vi "Write_To_File.vi"(8 "error in (no error)":errorcluster, 10 "Elevator Fleet":T1, 11 "refnum in":refnum<file>) -> (0 "error out":errorcluster, 3 "refnum out":refnum<file>)   [LabVIEW 2026]
uses:
  Controls/Elevator_Fleet.ctl
  Controls/Elevator_Status.ctl
  Controls/Door_Status_Enum.ctl
  Controls/Occupy_Status.ctl
  Controls/Floor_Status.ctl
  Controls/Motion_Status_Enum.ctl
  Controls/Car_Calls_Status.ctl
  Controls/Hall_Calls_Status.ctl
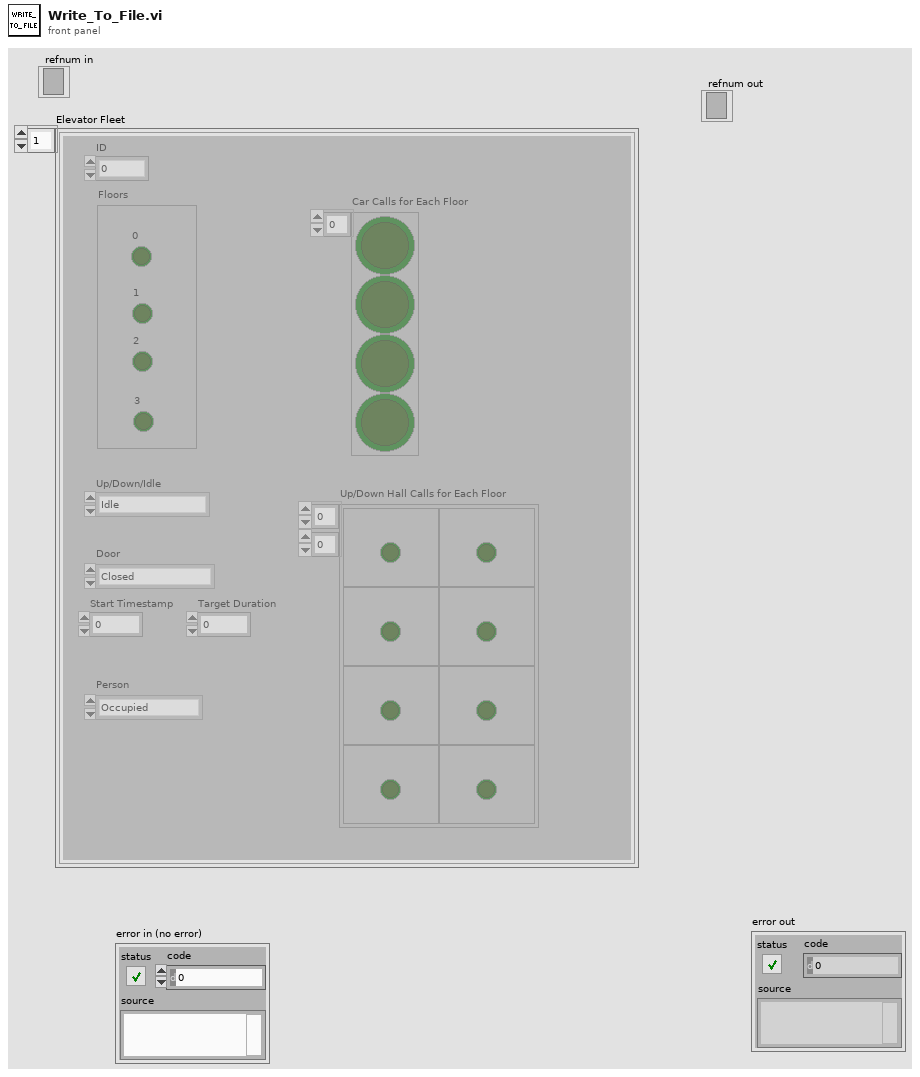
[diagram p1: front panel]
types:
  T1 = typedef "Elevator_Fleet.ctl" = T2[]
  T2 = typedef "Elevator_Status.ctl" = cluster{"Door":T3, "Person":T4, "Floors":T5, "Up/Down/Idle":T6, "Car Calls for Each Floor":T7, "Up/Down Hall Calls for Each Floor":T8, "ID":i32, "Start Timestamp":u32, "Target Duration":dbl}
  T3 = typedef "Door_Status_Enum.ctl" = enum16{"Closed", "Open", "Opening", "Closing"}
  T4 = typedef "Occupy_Status.ctl" = enum16{"Occupied", "Empty"}
  T5 = typedef "Floor_Status.ctl" = cluster{"0":bool, "1":bool, "2":bool, "3":bool}
  T6 = typedef "Motion_Status_Enum.ctl" = enum16{"Idle", "Up", "Down"}
  T7 = typedef "Car_Calls_Status.ctl" = bool[]
  T8 = typedef "Hall_Calls_Status.ctl" = cluster{bool}[][]
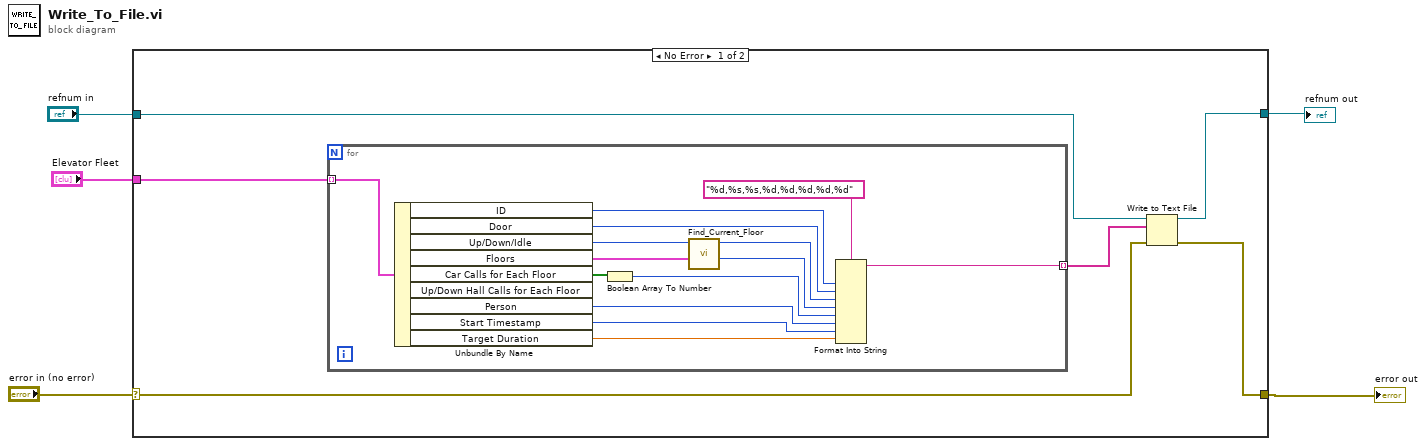
[diagram p0: block diagram]
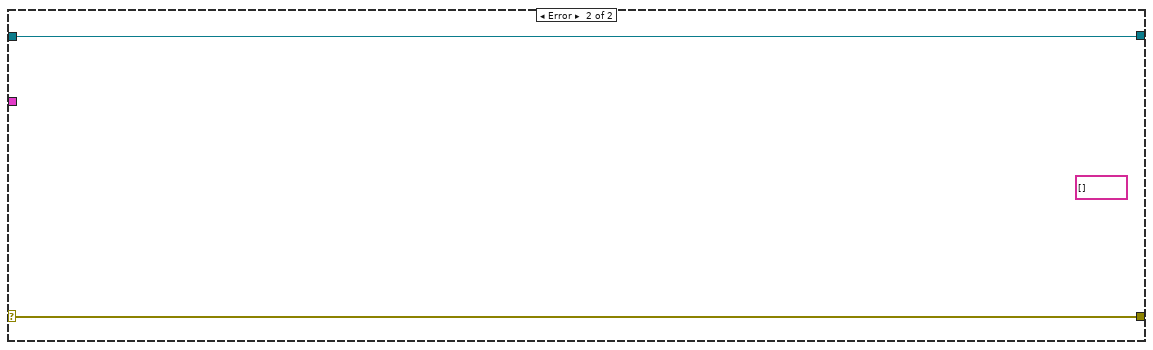
[diagram p2: hidden frame]
diagram:
  n1 = case shown="No Error" "error in (no error)" {
    selector: "error in (no error)" -> [w7 w26]
    tunnel: "Elevator Fleet" -> [w11 _]
    tunnel: [w6 w26] -> w3
    tunnel: "refnum in" -> [w8 w25]
    tunnel: [w10 w25] -> w1
    frame No Error {
      n2 = for {
        tunnel: w11 -> [w24] mode=indexing
        tunnel: [w12] -> w9 mode=indexing
        n3 = Unbundle By Name(w24) -> ("ID"=w20:i32, "Door"=w19:T3, "Up/Down/Idle"=w18:T6, "Floors"=w21:T5, "Car Calls for Each Floor"=w23:T7, "Person"=w15:T4, "Start Timestamp"=w14:u32, "Target Duration"=w13:dbl)  [unwired: 1 out]
        n4 = Boolean Array To Number(Boolean array=w23) -> (number=w16:u32)
        n5 = call "Find_Current_Floor.vi"("Floors"=w21) -> ("Current Floor"=w17:i32)  [unwired: 7 in, 3 out]
        n6 = Format Into String(format string="%d,%s,%s,%d,%d,%d,%d,%d", w20, w19, w18, w17, w16, w15, w14, w13) -> (resulting string=w12:string)  [unwired: 2 in, 1 out]
      }
      n7 = Write to Text File(file (use dialog)=w8, text=w9, error in=w7) -> (refnum out=w10:refnum<file>, error out=w6:errorcluster)  [unwired: 1 in, 1 out]
    }
    frame Error {
      (unwired) string[] []
    }
  }
  "error out" <- w3
  "refnum out" <- w1
